vi "Send Raw String.vi"(8 "error in (no error)":errorcluster, 10 "Cmd String":string, 11 "FW Arduino Control in":refnum<class "FW Arduino Control.lvclass">) -> (0 "error out":errorcluster, 3 "FW Arduino Control out":refnum<class "FW Arduino Control.lvclass">)   [LabVIEW 2024, in "FW Arduino Control.lvclass"]
uses:
  FW Arduino Control.lvclass
  C:/Development/Prime-RIMAS/Filter Wheel/Filter Wheel Object/Filter Wheel.lvclass
  FW Arduino Control.lvclass/FW Arduino Control.ctl
  Filter Wheel Object/Filter Wheel.lvclass
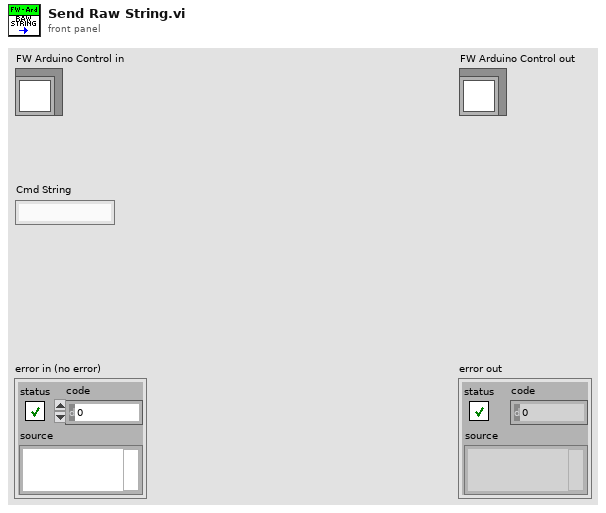
[diagram p1: front panel]
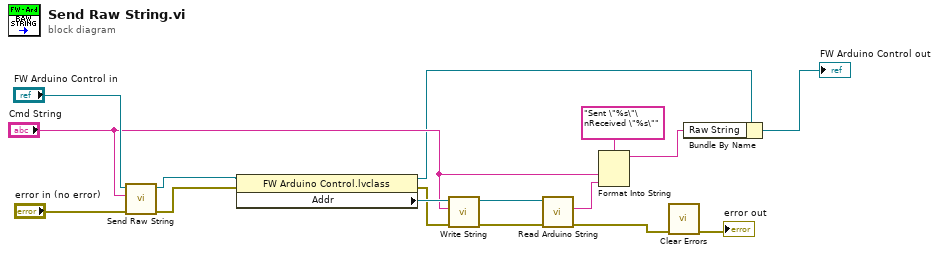
[diagram p0: block diagram]
diagram:
  n1 = call-parent "Send Raw String.vi"("error in (no error)"="error in (no error)", "Cmd String"="Cmd String", "Filter Wheel in"="FW Arduino Control in") -> ("error out"=w13:errorcluster, "Filter Wheel out"=w11:refnum<class "FW Arduino Control.lvclass">)  [unwired: 7 in]
  n2 = property class="FW Arduino Control.lvclass"(reference=w11, error in=w13) -> (reference out=w2:refnum<class "FW Arduino Control.lvclass">, error out=w12:errorcluster, "Addr"=w14:refnum<visa-resource-name>)
  n3 = call "Write String.vi"("error in (no error)"=w12, "String"="Cmd String", "VISA resource name"=w14) -> ("error out"=w9:errorcluster, "VISA resource name out"=w7:refnum<visa-resource-name>)  [unwired: 7 in]
  n4 = call "Read Arduino String.vi"("error in (no error)"=w9, "reference"=w7) -> ("error out"=w8:errorcluster, "response"=w3:string)  [unwired: 7 in, 1 out]
  n5 = Format Into String(format string="Sent \"%s\"\nReceived \"%s\"", "Cmd String", w3) -> (resulting string=w5:string)  [unwired: 2 in, 1 out]
  n6 = call <vilib>:"Clear Errors.vi"("error in (no error)"=w8) -> ("error out"=→"error out":errorcluster)  [unwired: 5 in, 1 out]
  n7 = Bundle By Name(cluster=w2, "Raw String"=w5) -> (→"FW Arduino Control out":refnum<class "FW Arduino Control.lvclass">)
